vi "SOFandEOF.vi"(8 "error in (no error)":errorcluster, 11 "Felica DOWN in":refnum<class "Felica DOWN.lvclass">) -> (0 "error out":errorcluster, 3 "Felica DOWN out":refnum<class "Felica DOWN.lvclass">, 5 "frame":u8[](array[numeric]))   [LabVIEW 2019, in "Felica DOWN.lvclass"]
uses:
  Felica DOWN.lvclass
  TypeDef/Store.ctl
  Felica DOWN.lvclass/Felica DOWN.ctl
  RFID system.lvclass
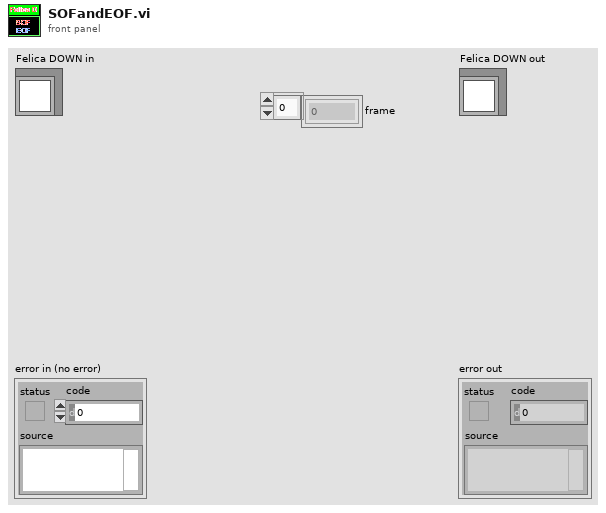
[diagram p1: front panel]
types:
  T1 = typedef "Store.ctl" = enum16{"envelope", "noise", "demSubCar", "CH_frame", "Decode", "demodulate", "in", "out", "sum", "subCarrier", "frame", "command", "encode", "modulate", "encode_UP", "modulate_up", "demod_up", "envelop_up", "sum_up", "out_up", "in_up"}
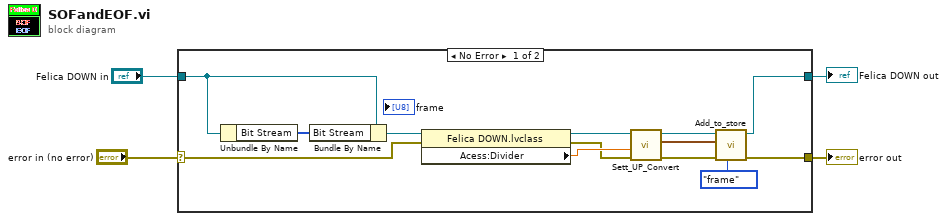
[diagram p0: block diagram]
diagram:
  n1 = case shown="No Error" "error in (no error)" {
    selector: "error in (no error)" -> [w6 w18]
    tunnel: [w11 w18] -> w3
    tunnel: "Felica DOWN in" -> [w10 w19]
    tunnel: [w12 w19] -> w1
    frame No Error {
      n2 = Unbundle By Name(w10) -> ("Bit Stream"=w9:u8[])
      n3 = Bundle By Name(cluster=w10, "Bit Stream"=w9) -> (w17:refnum<class "Felica DOWN.lvclass">)
      n4 = property class="Felica DOWN.lvclass"(reference=w17, error in=w6) -> (reference out=w8:refnum<class "Felica DOWN.lvclass">, error out=w5:errorcluster, "Acess:Divider"=w7:dbl)
      n5 = call-dynamic "Sett_UP_Convert.vi"("error in (no error)"=w5, "Divider(1)"=w7, "Felica DOWN in"=w8) -> ("error out"=w14:errorcluster, "Waveform"=w15:waveform(dbl), "Felica DOWN out"=w16:refnum<class "Felica DOWN.lvclass">)  [unwired: 6 in]
      n6 = call "Add_to_store.vi"("Store"=Store."frame", "error in (no error)"=w14, "Waveform"=w15, "RFID system in"=w16) -> ("error out"=w11:errorcluster, "RFID system out"=w12:refnum<class "Felica DOWN.lvclass">)  [unwired: 6 in]
    }
    frame Error {
    }
  }
  "error out" <- w3
  "Felica DOWN out" <- w1
